vi "Run Panel VI.vi"(8 "error in (no error)":errorcluster, 11 "Panel in":refnum<class "Panel.lvclass">) -> (0 "error out":errorcluster, 3 "Panel out":refnum<class "Panel.lvclass">)   [LabVIEW 2020, in "OOPanel.lvlib" / "Panel.lvclass"]
uses:
  Panel.lvclass
  Panel.lvclass/Panel.ctl
  Visibility State.ctl
  <vilib>/Utility/error.llb/Error Cluster From Error Code.vi
  <vilib>/ErrorRing/Error Ring.xnode
  OOPanel.lvlib
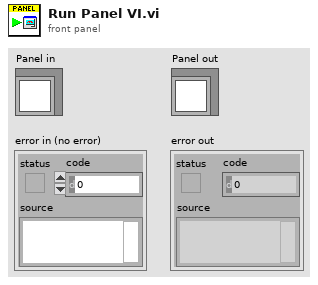
[diagram p1: front panel]
types:
  T1 = typedef "OOPanel.lvlib/Visibility State.ctl" = enum16{"Idle", "Closed", "Hidden", "Visible", "Subpanel"}
  T2 = enum32{"Invalid", "Standard", "Closed", "Hidden", "Minimized", "Maximized"}
  T3 = typedef "OOPanel.lvlib/Panel.lvclass/Ref Data.ctl" = cluster{"Panel Ref":refnum<vi>, "SubPanel":refnum<vi>, "Close":bool, "Running":bool, "State":T4}
  T4 = typedef "OOPanel.lvlib/Panel.lvclass/Visibility State.ctl" = enum16{"Idle", "Closed", "Hidden", "Visible", "Subpanel"}
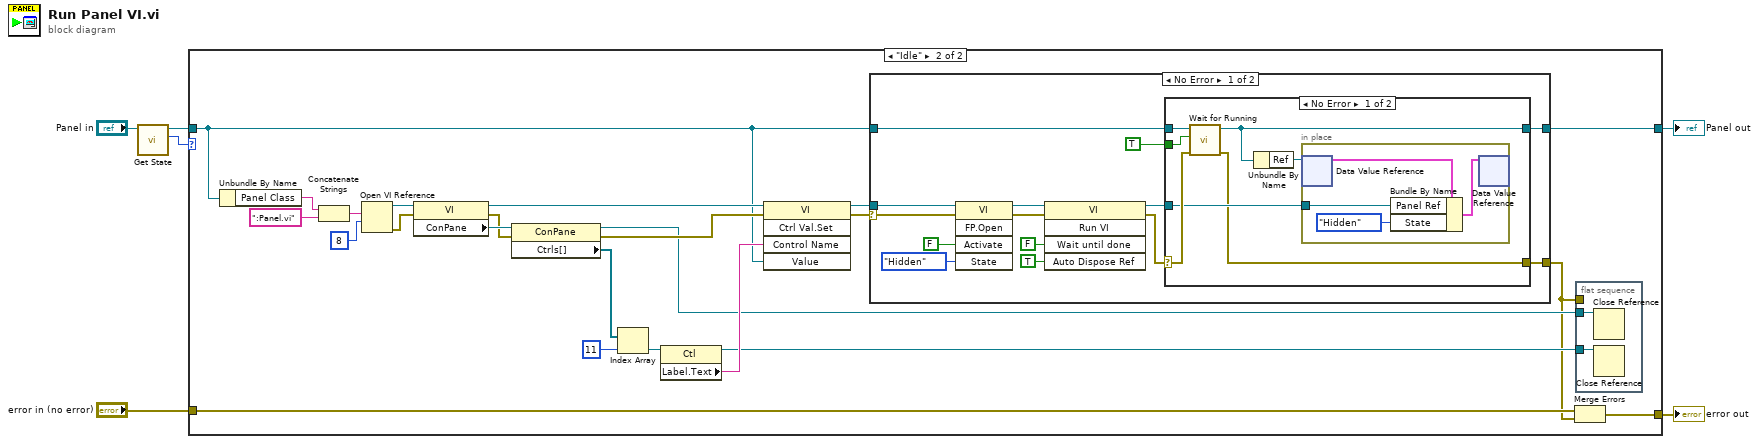
[diagram p0: block diagram]
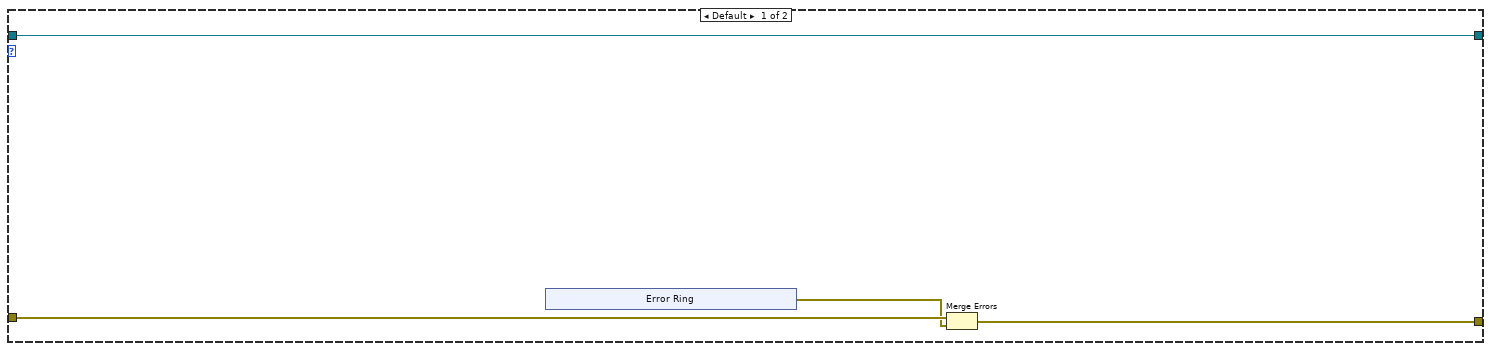
[diagram p2: hidden frame]
diagram:
  n1 = call "Get State.vi"("Panel in"="Panel in") -> ("State"=w1:T1, "Panel out"=w2:refnum<class "Panel.lvclass">)  [unwired: 8 in, 1 out]
  n2 = case shown="\"Idle\"" w1 {
    tunnel: "error in (no error)" -> [w9 w37]
    tunnel: [w10 w21] -> w5
    tunnel: [w7 w20] -> w4
    tunnel: w2 -> [w10 w16]
    frame Default {
      n3 = xnode "Error Ring"() -> ("error out"=w8:errorcluster)
      n4 = Merge Errors(w9, w8) -> (w7:errorcluster)
    }
    frame "Idle" {
      n5 = Unbundle By Name(w16) -> ("Panel Class"=w15:string)
      n6 = Concatenate Strings(w15, ":Panel.vi" ("string")) -> (w35:string)
      n7 = Open VI Reference(vi path=w35, options=8) -> (vi reference=w34:refnum<vi>, error out=w33:errorcluster)  [unwired: 4 in]
      n8 = property class="VI"(reference=w34, error in=w33) -> (reference out=w29:refnum<vi>, error out=w27:errorcluster, "ConPane"=w32:refnum<vi>)
      n9 = property class="ConPane"(reference=w32, error in=w27) -> (reference out=w22:refnum<vi>, error out=w26:errorcluster, "Ctrls[]"=w31:refnum<vi>[])
      n10 = Index Array(array=w31, index=11) -> (element=w30:refnum<vi>)
      n11 = property class="Ctl"(reference=w30) -> (reference out=w23:refnum<vi>, "Label.Text"=w28:string)  [unwired: 1 in, 1 out]
      n12 = invoke class="VI" method="Ctrl Val.Set"(reference=w29, error in=w26, "Control Name"=w28, "Value"=w16) -> (reference out=w18:refnum<vi>, error out=w24:errorcluster)  [unwired: 1 in, 3 out]
      n13 = case shown="No Error" w24 {
        selector: w24 -> [w44 w67]
        tunnel: w18 -> [w45 _]
        tunnel: [w46 w67] -> w19
        tunnel: w16 -> [w50 w68]
        tunnel: [w49 w68] -> w21
        frame No Error {
          n14 = invoke class="VI" method="FP.Open"(reference=w45, error in=w44, "Activate"=FALSE ("Activate?"), "State"=T2."Hidden") -> (reference out=w41:refnum<vi>, error out=w40:errorcluster)  [unwired: 1 in, 3 out]
          n15 = invoke class="VI" method="Run VI"(reference=w41, error in=w40, "Wait until done"=FALSE ("Wait Until Done"), "Auto Dispose Ref"=TRUE ("Auto Dispose Reference")) -> (reference out=w51:refnum<vi>, error out=w47:errorcluster)  [unwired: 1 in, 3 out]
          n16 = case shown="No Error" w47 {
            selector: w47 -> [w56 w66]
            tunnel: w51 -> [w55 _]
            tunnel: w50 -> [w59 w65]
            tunnel: [w58 w65] -> w49
            tunnel: TRUE ("Running") -> [w57 _]
            tunnel: [w54 w66] -> w46
            frame No Error {
              n17 = call "Wait for Running.vi"("error in (no error)"=w56, "Running"=w57, "Panel in"=w59) -> ("error out"=w54:errorcluster, "Panel out"=w58:refnum<class "Panel.lvclass">)  [unwired: 7 in]
              n18 = Unbundle By Name(w58) -> ("Ref"=w60:refnum<data-value>)
              n19 = in-place {
                in-place-border: w55 -> [w61]
                n20 = in-place-dvr #1(w60) -> (w64:T3)  [unwired: 1 out]
                n21 = Bundle By Name(cluster=w64, "Panel Ref"=w61, "State"=Visibility_State."Hidden") -> (w63:T3)
                n22 = in-place-dvr #1(w63) -> ()  [unwired: 2 out]
              }
            }
            frame Error {
            }
          }
        }
        frame Error {
        }
      }
      n23 = Merge Errors(w37, w19) -> (w20:errorcluster)
      n24 = flat-sequence {
        tunnel: w23 -> [w39]
        tunnel: [w38] -> _
        tunnel: w22 -> [w38]
        tunnel: w19 -> [_]
        frame #0 {
          n25 = Close Reference(reference=w38) -> ()  [unwired: 1 in, 1 out]
          n26 = Close Reference(reference=w39) -> ()  [unwired: 1 in, 1 out]
        }
      }
    }
  }
  "error out" <- w4
  "Panel out" <- w5
